vi "TDMS Report_Init.vi"(8 "error in (no error)":errorcluster) -> (0 "error out":errorcluster, 3 "TDMS Report out":refnum<class "TDMS Report - Solution.lvclass">)   [LabVIEW 2011, in "TDMS Report - Solution.lvclass"]
doc: "Part of the solution for the TDMS Report Object. This creates a TDMS object.\n\nAAL 9/09"
uses:
  TDMS Report - Solution.lvclass
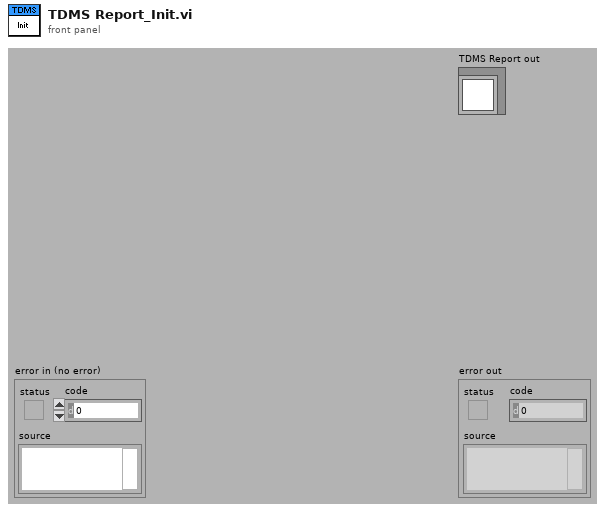
[diagram p1: front panel]
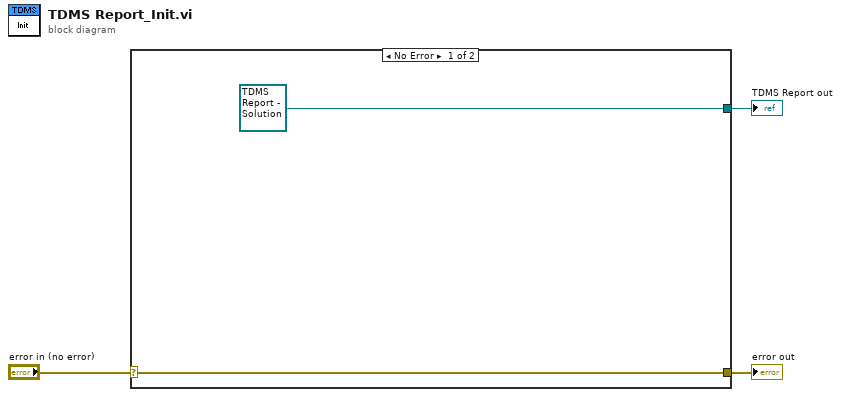
[diagram p0: block diagram]
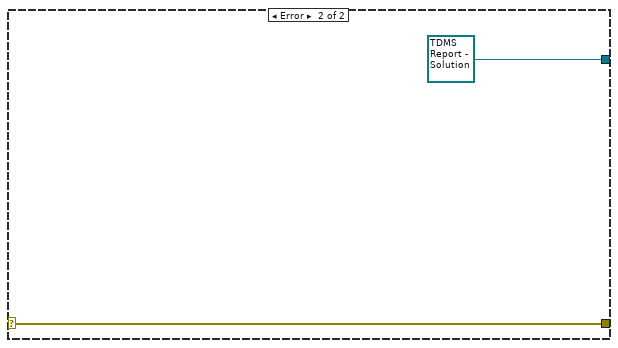
[diagram p2: hidden frame]
diagram:
  n1 = case shown="No Error" "error in (no error)" {
    selector: "error in (no error)" -> [w4 w7]
    tunnel: [w4 w7] -> w2
    tunnel: [refnum<class "TDMS Report - Solution.lvclass"> refnum ("TXT_Report.lvclass") refnum<class "TDMS Report - Solution.lvclass"> refnum ("TXT_Report.lvclass")] -> w1
    frame No Error {
    }
    frame Error {
    }
  }
  "error out" <- w2
  "TDMS Report out" <- w1
